vi "global-refs.vi"(0 "ZuoQian":T4, 1 "Robot":refnum<vi>, 5 "ZuoHou":T1, 7 "Read?":bool=TRUE, 9 "YouQian":T3, 11 "YouHou":T2, 12 "Body":refnum<vi>) -> (3 "RobotRef":refnum<vi>, 4 "ZuoQianRef":T4, 6 "ZuoHouRef":T1, 10 "YouQianRef":T3, 14 "BodyRef":refnum<vi>, 15 "YouHouRef":T2)   [LabVIEW 2013]
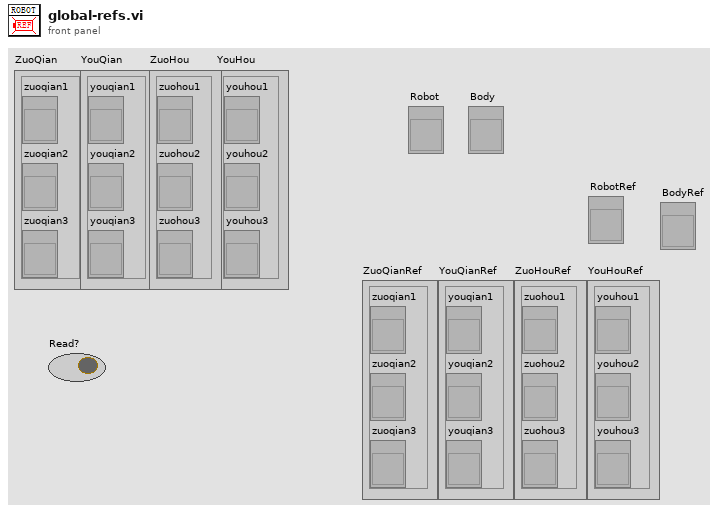
[diagram p1: front panel]
types:
  T1 = cluster{"zuohou1":refnum<vi>, "zuohou2":refnum<vi>, "zuohou3":refnum<vi>}
  T2 = cluster{"youhou1":refnum<vi>, "youhou2":refnum<vi>, "youhou3":refnum<vi>}
  T3 = cluster{"youqian1":refnum<vi>, "youqian2":refnum<vi>, "youqian3":refnum<vi>}
  T4 = cluster{"zuoqian1":refnum<vi>, "zuoqian2":refnum<vi>, "zuoqian3":refnum<vi>}
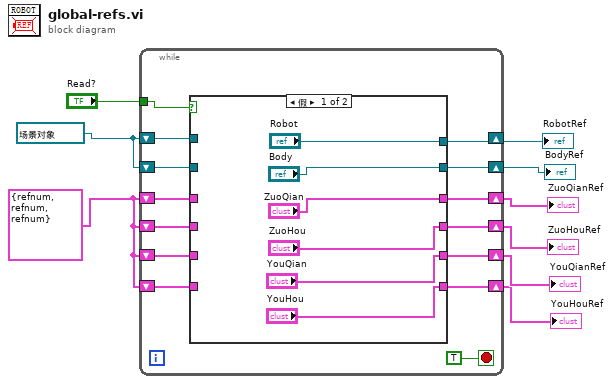
[diagram p0: block diagram]
diagram:
  w8 = T1 {"zuohou1"=refnum, "zuohou2"=refnum, "zuohou3"=refnum} ("ZuoHou")
  w7 = refnum<vi> refnum ("Body")
  n1 = while {
    shift-right: [w19] -> w4
    shift-left: w8 -> [w13]
    shift-right: [w18] -> w3
    shift-left: w8 -> [w12]
    shift-right: [w17] -> w2
    shift-left: w8 -> [w11]
    shift-right: [w16] -> w1
    shift-left: w8 -> [w10]
    shift-right: [w20] -> w5
    shift-left: w7 -> [w14]
    shift-right: [w21] -> w6
    shift-left: w7 -> [w15]
    tunnel: "Read?" -> [w22]
    stop <- TRUE stop-if-true
    n2 = case shown="假" w22 {
      tunnel: ["Robot" w35] -> w21
      tunnel: ["Body" w34] -> w20
      tunnel: ["ZuoQian" w33] -> w19
      tunnel: ["ZuoHou" w32] -> w18
      tunnel: ["YouQian" w31] -> w17
      tunnel: ["YouHou" w30] -> w16
      tunnel: w15 -> [_ w35]
      tunnel: w14 -> [_ w34]
      tunnel: w13 -> [_ w33]
      tunnel: w12 -> [_ w32]
      tunnel: w11 -> [_ w31]
      tunnel: w10 -> [_ w30]
      frame False {
      }
      frame True {
      }
    }
  }
  "ZuoQianRef" <- w4
  "YouQianRef" <- w2
  "YouHouRef" <- w1
  "ZuoHouRef" <- w3
  "RobotRef" <- w6
  "BodyRef" <- w5
